vi "JL_Scaling Factor.vi"(8 "Error":errorcluster, 9 "Scalling":T2, 10 "Scaling Type":T3=enum."Scale Voltage", 11 "Desired Value Out":dbl) -> (0 "Error Out":errorcluster, 2 "Slope and Intercept":cluster{"Voltage Scalling":T1} {"Voltage Scalling"."Slope" format="%#_11g"}, 3 "Analog Value Out":dbl)   [LabVIEW 2023]
doc: "Utility to convert raw values from the analog input card to actual values."
uses:
  Controls/ENUM_JL Scaling Factor_.ctl
  Controls/Cluster_JL Scaling Control.ctl
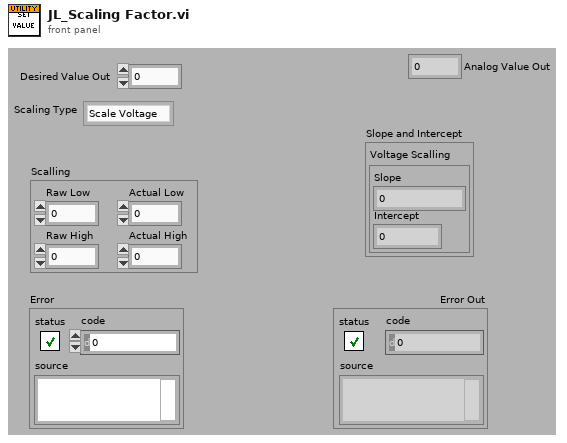
[diagram p1: front panel]
types:
  T1 = typedef "Cluster_JL Scaling Control.ctl" = cluster{"Slope":dbl, "Intercept":dbl}
  T2 = cluster{"Raw Low ":dbl, "Raw High":dbl, "Actual Low":dbl, "Actual High":dbl}
  T3 = typedef "ENUM_JL Scaling Factor_.ctl" = enum16{"Init", "Scale Voltage", "Flush Slope"}
  T4 = cluster{"Calibrate?":bool, "Scalling In ":cluster{"Raw Low ":dbl, "Raw High":dbl, "Actual Low":dbl, "Actual High":dbl}}
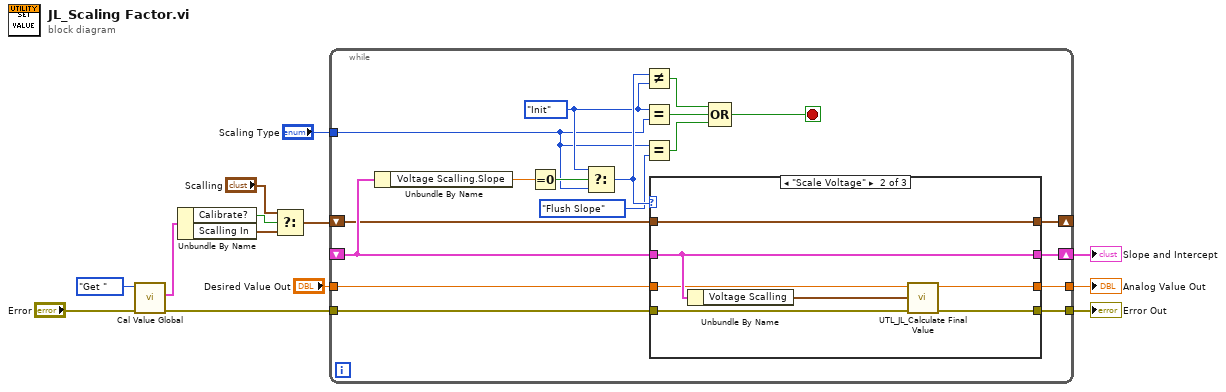
[diagram p0: block diagram]
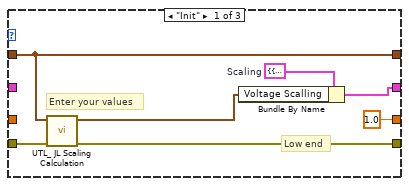
[diagram p2: hidden frame]
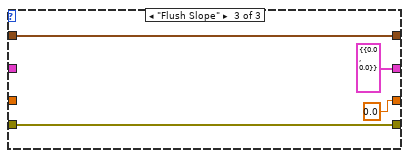
[diagram p3: hidden frame]
diagram:
  n1 = call "Cal Value Global.vi"("error in (no error)"="Error", "Action"=enum16{"Set", "Get "}."Get ") -> ("error out"=w4:errorcluster, "Cal  Out"=w2:T4)  [unwired: 8 in]
  n2 = Unbundle By Name(w2) -> ("Calibrate?"=w1:bool, "Scalling In"=w3:T2)
  n3 = Select(t="Scalling", s=w1, f=w3) -> (s? t:f=w7:T2)
  n4 = while {
    tunnel: [w31] -> w10
    tunnel: "Desired Value Out" -> [w30]
    tunnel: "Scaling Type" -> [w16]
    tunnel: w4 -> [w29]
    tunnel: [w28] -> w11
    shift-right: [w27] -> w9
    shift-left: _ -> [w26]
    shift-right: [w18] -> _
    shift-left: w7 -> [w19]
    stop <- w22 stop-if-true
    w20 = ENUM_JL_Scaling_Factor_."Init" ("t")
    n5 = Unbundle By Name(w26) -> ("Voltage Scalling.Slope"=w24:dbl)
    n6 = Equal To 0?(x=w24) -> (x = 0?=w23:bool)
    n7 = Select(t=w20, s=w23, f=w16) -> (s? t:f=w25:T3)
    n8 = Not Equal?(x=w25, y=w20) -> (x != y?=w21:bool)
    n9 = Equal?(x=w20, y=w16) -> (x = y?=w17:bool)
    n10 = Equal?(x=w16, y=ENUM_JL_Scaling_Factor_."Flush Slope") -> (x = y?=w14:bool)
    n11 = case shown="\"Scale Voltage\"" w25 {
      tunnel: [1.0 ("Analog Value") w41 0.0 ("Analog Value Out")] -> w31
      tunnel: w30 -> [_ w40 _]
      tunnel: w29 -> [w33 w44 w49]
      tunnel: [w32 w43 w49] -> w28
      tunnel: [w36 w45 cluster{"Voltage Scalling":T1} {"Voltage Scalling"={"Slope"=0.0, "Intercept"=0.0}}] -> w27
      tunnel: w26 -> [_ w45 _]
      tunnel: w19 -> [w34 w39 w46]
      tunnel: [w34 w39 w46] -> w18
      frame "Init" {
        w37 = cluster{"Voltage Scalling":T1} {"Voltage Scalling"={"Slope"=0.0, "Intercept"=0.0}}  # Scaling
        # "Low end"
        # "Enter your values"
        n12 = call "UTL_ JL Scaling Calculation.vi"("Error"=w33, "Scaling Parameters"=w34) -> ("Error Out"=w32:errorcluster, "Scaling Factors Out"=w35:T1)  [unwired: 8 in]
        n13 = Bundle By Name(cluster=w37, "Voltage Scalling"=w35) -> (w36:cluster{"Voltage Scalling":T1})
      }
      frame "Scale Voltage" {
        n14 = Unbundle By Name(w45) -> ("Voltage Scalling"=w42:T1)
        n15 = call "UTL_JL_Calculate Final Value.vi"("Error"=w44, "Voltage Scalling"=w42, "Analog Value"=w40) -> ("Error Out"=w43:errorcluster, "Analog Value Out"=w41:dbl)  [unwired: 7 in]
      }
      frame "Flush Slope" {
      }
    }
    n16 = Compound Arithmetic op=OR(w21, w17, w14) -> (w22:bool)
  }
  "Analog Value Out" <- w10
  "Error Out" <- w11
  "Slope and Intercept" <- w9
